vi "Compose TOML String.vi"(8 "error in (no error)":errorcluster, 11 "Value":T1) -> (0 "error out":errorcluster, 3 "String":string)   [LabVIEW 2019, in "BlueTOMLSerializer.lvlib"]
uses:
  BlueTOMLSerializer.lvlib
  TOML Value.ctl
  Compose Data.ctl
  Value.ctl
  Value Type.ctl
  Key-Value Pair.ctl
  <vilib>/regexp/Match Regular Expression.xnode
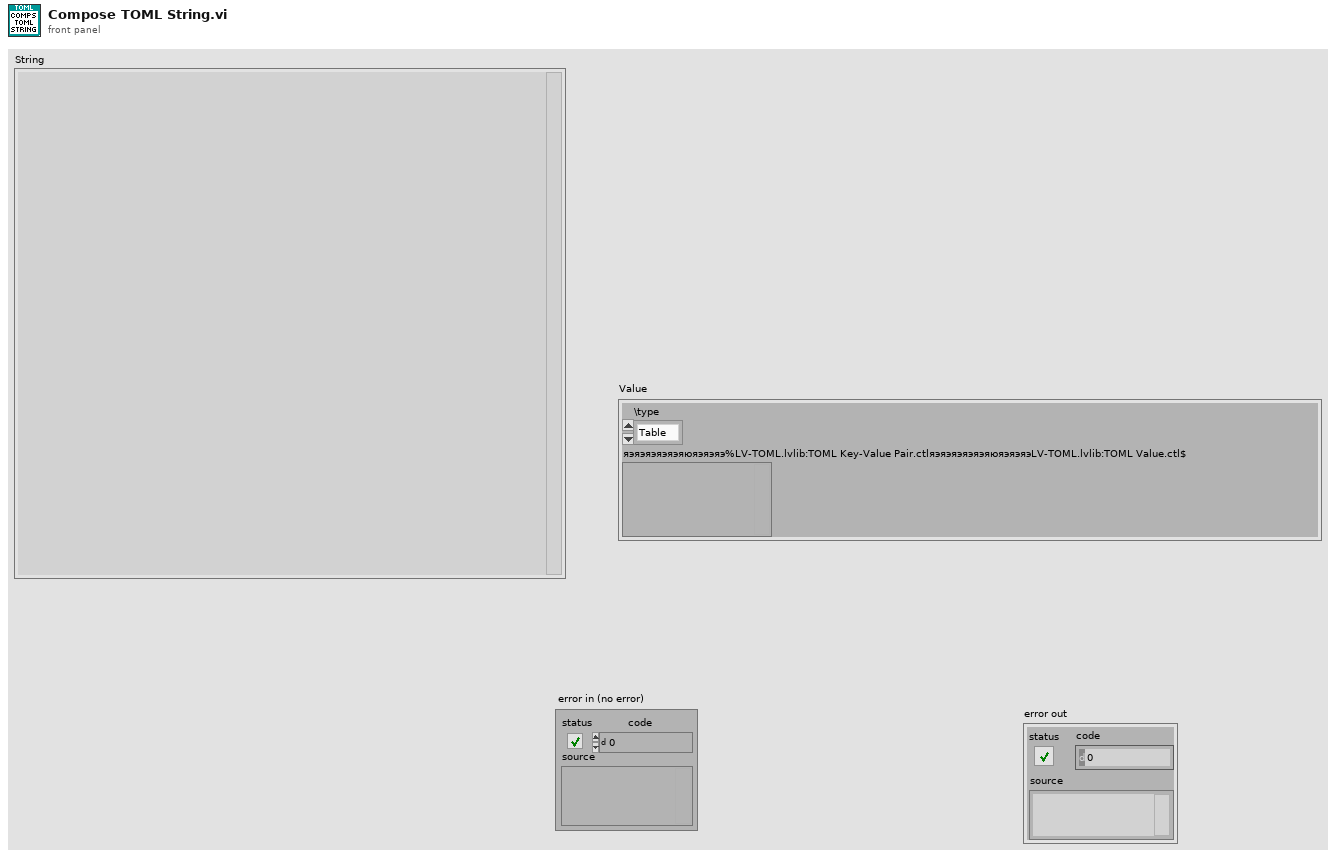
[diagram p1: front panel]
types:
  T1 = typedef "BlueTOMLSerializer.lvlib/TOML Value.ctl" = cluster{"\\type":enum16{"Table", "Array", "String", "Integer", "Float", "Boolean", "Offset Date-Time", "Local Date-Time", "Local Date", "Local Time"}, "яэяэяэяэяэяюяэяэяэ%LV-TOML.lvlib:TOML Key-Value Pair.ctlяэяэяэяэяэяюяэяэяэLV-TOML.lvlib:TOML Value.ctl$":variant}
  T2 = typedef "BlueTOMLSerializer.lvlib/Compose Data.ctl" = cluster{"Value":T3, "Prepend":string, "Append":string, "Inline":bool, "Name":string}
  T3 = typedef "BlueTOMLSerializer.lvlib/Value.ctl" = cluster{"Type":T4, "Value":variant}
  T4 = typedef "BlueTOMLSerializer.lvlib/Value Type.ctl" = enum16{"Table", "Array", "String", "Integer", "Float", "Boolean", "Offset Date-Time", "Local Date-Time", "Local Date", "Local Time"}
  T5 = typedef "BlueTOMLSerializer.lvlib/Key-Value Pair.ctl" = cluster{"Key":string, "Value":T3}
  T6 = enum16{"Table", "Array", "String", "Integer", "Float", "Boolean", "Offset Date-Time", "Local Date-Time", "Local Date", "Local Time"}
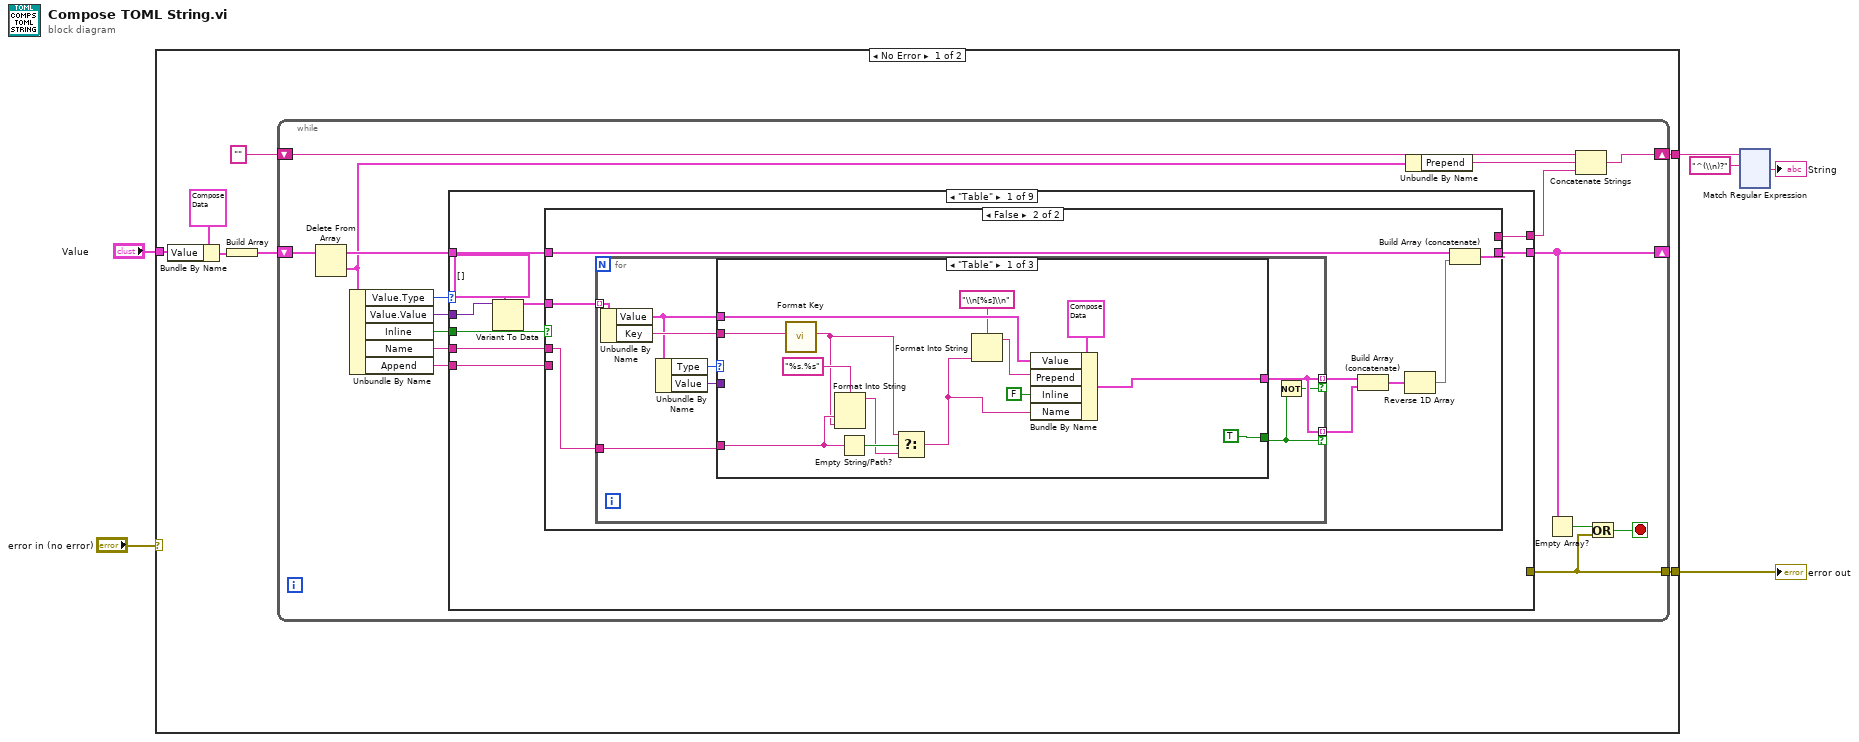
[diagram p0: block diagram]
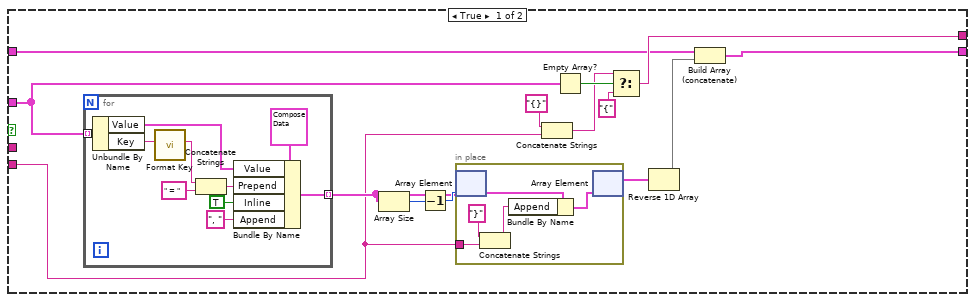
[diagram p2: hidden frame]
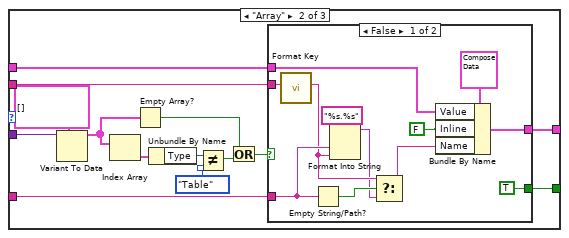
[diagram p3: hidden frame]
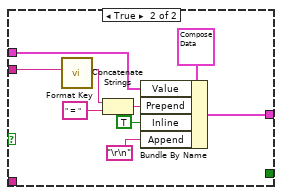
[diagram p4: hidden frame]
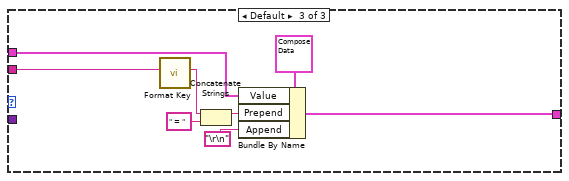
[diagram p5: hidden frame]
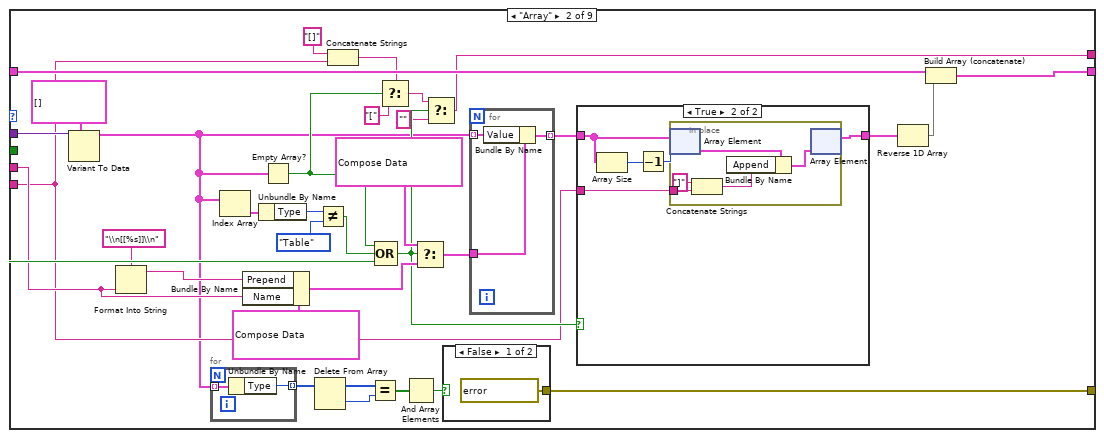
[diagram p6: hidden frame]
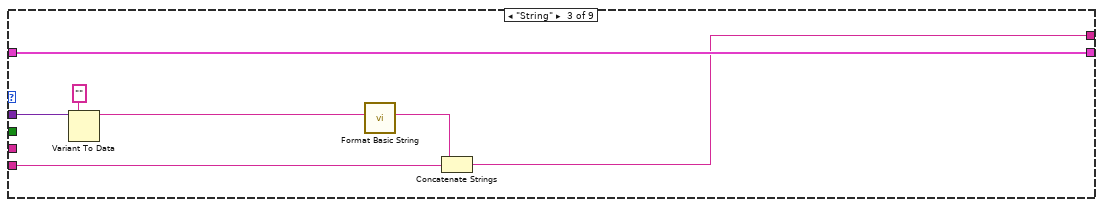
[diagram p9: hidden frame]
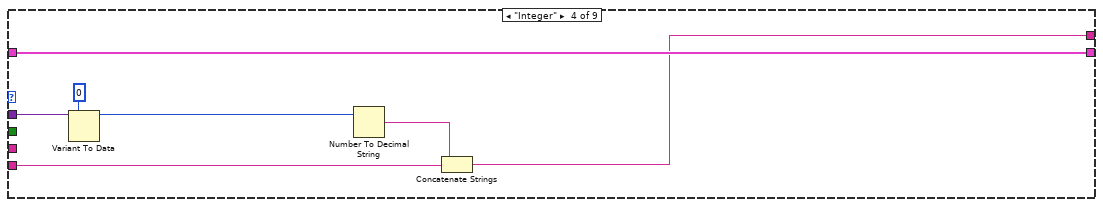
[diagram p10: hidden frame]
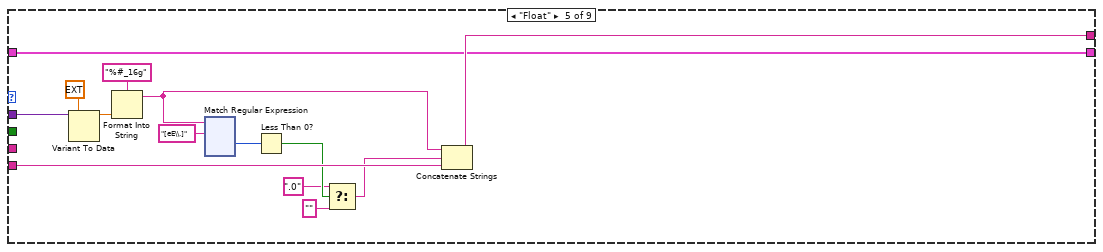
[diagram p11: hidden frame]
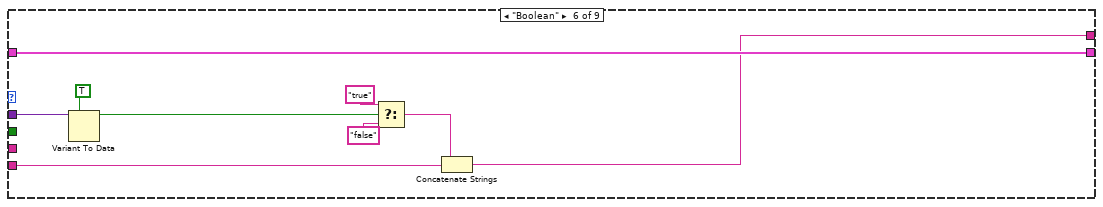
[diagram p12: hidden frame]
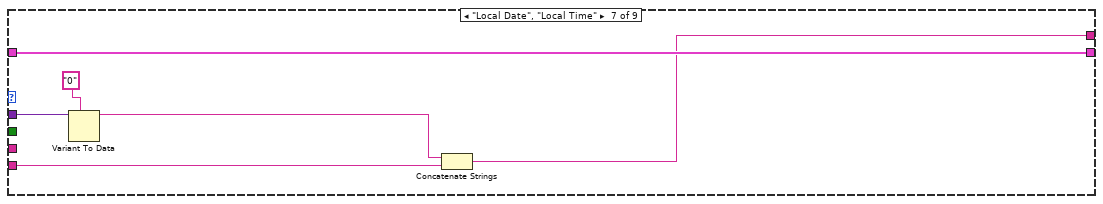
[diagram p13: hidden frame]
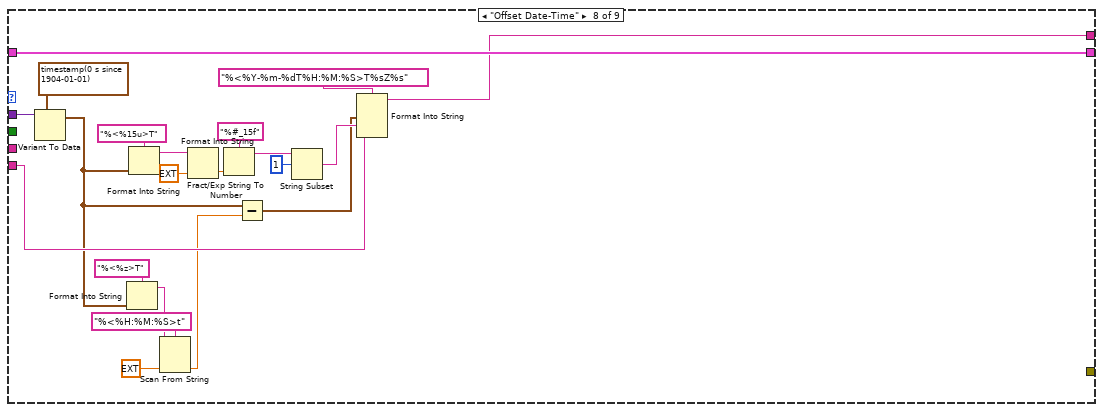
[diagram p14: hidden frame]
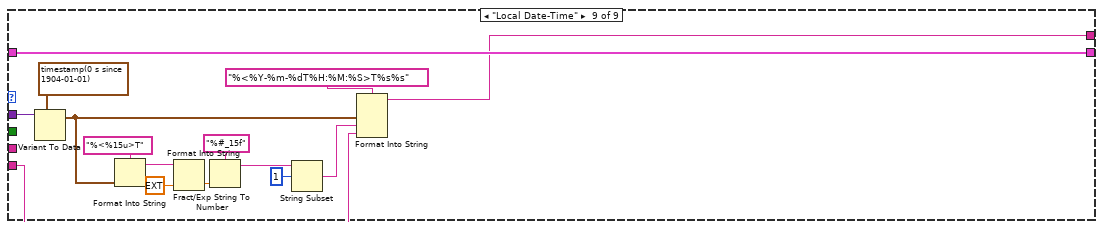
[diagram p15: hidden frame]
diagram:
  n1 = case shown="No Error" "error in (no error)" {
    selector: "error in (no error)" -> [_ w387]
    tunnel: "Value" -> [w10 _]
    tunnel: [w8 _] -> w1
    tunnel: [w7 w387] -> w4
    frame No Error {
      n2 = Bundle By Name(cluster=T2 {"Value"={"Type"=enum."Table", "Value"=variant}, "Prepend"="", "Append"="", "Inline"=FALSE, "Name"=""}, "Value"=w10) -> (w9:T2)
      n3 = Build Array(w9) -> (w12:T2[])
      n4 = while {
        shift-right: [w20] -> w8
        shift-left: "" -> [w23]
        shift-right: [w21] -> _
        shift-left: w12 -> [w29]
        tunnel: [w14] -> w7
        stop <- w15 stop-if-true
        n5 = Delete From Array(array=w29) -> (deleted portion=w18:T2, array with subset deleted=w26:T2[])  [unwired: 2 in]
        n6 = Unbundle By Name(w18) -> ("Value.Type"=w28:T4, "Value.Value"=w27:variant, "Inline"=w25:bool, "Name"=w24:string, "Append"=w16:string)
        n7 = case shown="\"Table\"" w28 {
          tunnel: w27 -> [w35 w176 w199 w206 w221 w344 w350 w370 w385]
          tunnel: w26 -> [w38 w163 w200 w207 w216 w342 w348 w371 w386]
          tunnel: [w37 w149 w200 w207 w216 w342 w348 w371 w386] -> w21
          tunnel: w25 -> [w36 w170 _ _ _ _ _ _ _]
          tunnel: w24 -> [w32 w152 _ _ _ _ _ _ _]
          tunnel: [w30 w156 w194 w201 w218 w336 w345 w362 w379] -> w19
          tunnel: w16 -> [w31 w150 w195 w204 w219 w343 w349 w363 w380]
          tunnel: [_ w142 _ _ _ _ _ _ _] -> w14
          frame "Table" {
            n8 = Variant To Data(type=T5[] [], Variant=w35) -> (data=w33:T5[])  [unwired: 1 in, 1 out]
            n9 = case shown="False" w36 {
              tunnel: w38 -> [w42 w75]
              tunnel: [w41 w74] -> w37
              tunnel: w33 -> [w49 w71]
              tunnel: w32 -> [_ w73]
              tunnel: w31 -> [w46 _]
              tunnel: [w45 _] -> w30
              frame True {
                n10 = for {
                  tunnel: w49 -> [w67] mode=indexing
                  tunnel: [w59] -> w50 mode=indexing
                  n11 = Unbundle By Name(w67) -> ("Value"=w64:T3, "Key"=w66:string)
                  n12 = call "Format Key.vi"("Key String"=w66) -> ("Formatted Key"=w62:string)  [unwired: 10 in]
                  n13 = Concatenate Strings(w62, " = " ("string")) -> (w63:string)
                  n14 = Bundle By Name(cluster=T2 {"Value"={"Type"=enum."Table", "Value"=variant}, "Prepend"="", "Append"="", "Inline"=FALSE, "Name"=""}, "Value"=w64, "Prepend"=w63, "Inline"=TRUE, "Append"=", ") -> (w59:T2)
                }
                n15 = Array Size(array=w50) -> (size(s)=w52:i32)
                n16 = Decrement(x=w52) -> (x-1=w51:i32)
                n17 = in-place {
                  in-place-border: w46 -> [w53]
                  n18 = in-place-array #1(w50, w51) -> (w57:T2)
                  n19 = Concatenate Strings("}" ("Prepend"), w53) -> (w54:string)
                  n20 = Bundle By Name(cluster=w57, "Append"=w54) -> (w56:T2)
                  n21 = in-place-array #1(w56) -> (w44:T2[])  [unwired: 1 out]
                }
                n22 = Concatenate Strings("{}" ("Prepend"), w46) -> (w39:string)
                n23 = Empty Array?(array=w49) -> (empty?=w48:bool)
                n24 = Select(t=w39, s=w48, f="{" ("t")) -> (s? t:f=w45:string)
                n25 = Reverse 1D Array(array=w44) -> (reversed array=w43:T2[])
                n26 = Build Array (concatenate)(w42, w43) -> (w41:T2[])
              }
              frame False {
                n27 = for {
                  tunnel: w71 -> [w84] mode=indexing
                  tunnel: [w78] -> w69 mode=indexing if=w77
                  tunnel: w73 -> [w80]
                  tunnel: [w78] -> w68 mode=indexing if=w76
                  n28 = Unbundle By Name(w84) -> ("Value"=w82:T3, "Key"=w83:string)
                  n29 = Unbundle By Name(w82) -> ("Type"=w81:T4, "Value"=w79:variant)
                  n30 = case shown="\"Table\"" w81 {
                    tunnel: w83 -> [w98 w112 w137]
                    tunnel: [w95 w111 w134] -> w78
                    tunnel: w82 -> [w94 w110 w136]
                    tunnel: w80 -> [w90 w109 _]
                    tunnel: w79 -> [_ w101 _]
                    tunnel: [TRUE w99 _] -> w76
                    frame "Table" {
                      n31 = call "Format Key.vi"("Key String"=w98) -> ("Formatted Key"=w88:string)  [unwired: 10 in]
                      n32 = Format Into String(format string="%s.%s", w90, w88) -> (resulting string=w87:string)  [unwired: 2 in, 1 out]
                      n33 = Empty String/Path?(string/path=w90) -> (empty?=w89:bool)
                      n34 = Select(t=w88, s=w89, f=w87) -> (s? t:f=w86:string)
                      n35 = Format Into String(format string="\\n[%s]\\n", w86) -> (resulting string=w91:string)  [unwired: 2 in, 1 out]
                      n36 = Bundle By Name(cluster=T2 {"Value"={"Type"=enum."Table", "Value"=variant}, "Prepend"="", "Append"="", "Inline"=FALSE, "Name"=""}, "Value"=w94, "Prepend"=w91, "Inline"=FALSE, "Name"=w86) -> (w95:T2)
                    }
                    frame "Array" {
                      n37 = Variant To Data(type=T3[] [], Variant=w101) -> (data=w104:T3[])  [unwired: 1 in, 1 out]
                      n38 = Index Array(array=w104) -> (element=w106:T3)  [unwired: 1 in]
                      n39 = Empty Array?(array=w104) -> (empty?=w108:bool)
                      n40 = Unbundle By Name(w106) -> ("Type"=w105:T4)
                      n41 = Not Equal?(x=w105, y=T6."Table") -> (x != y?=w107:bool)
                      n42 = Or(x=w108, y=w107) -> (x .or. y?=w100:bool)
                      n43 = case shown="False" w100 {
                        tunnel: w112 -> [w119 w127]
                        tunnel: [w122 w125] -> w111
                        tunnel: w110 -> [w121 w128]
                        tunnel: w109 -> [w118 _]
                        tunnel: [TRUE _] -> w99
                        frame False {
                          n44 = call "Format Key.vi"("Key String"=w119) -> ("Formatted Key"=w116:string)  [unwired: 10 in]
                          n45 = Empty String/Path?(string/path=w118) -> (empty?=w117:bool)
                          n46 = Format Into String(format string="%s.%s", w118, w116) -> (resulting string=w115:string)  [unwired: 2 in, 1 out]
                          n47 = Select(t=w116, s=w117, f=w115) -> (s? t:f=w114:string)
                          n48 = Bundle By Name(cluster=T2 {"Value"={"Type"=enum."Table", "Value"=variant}, "Prepend"="", "Append"="", "Inline"=FALSE, "Name"=""}, "Value"=w121, "Inline"=FALSE, "Name"=w114) -> (w122:T2)
                        }
                        frame True {
                          n49 = call "Format Key.vi"("Key String"=w127) -> ("Formatted Key"=w131:string)  [unwired: 10 in]
                          n50 = Concatenate Strings(w131, " = " ("string")) -> (w132:string)
                          n51 = Bundle By Name(cluster=T2 {"Value"={"Type"=enum."Table", "Value"=variant}, "Prepend"="", "Append"="", "Inline"=FALSE, "Name"=""}, "Value"=w128, "Prepend"=w132, "Inline"=TRUE, "Append"="\r\n") -> (w125:T2)
                        }
                      }
                    }
                    frame Default {
                      n52 = call "Format Key.vi"("Key String"=w137) -> ("Formatted Key"=w139:string)  [unwired: 10 in]
                      n53 = Concatenate Strings(w139, " = " ("string")) -> (w140:string)
                      n54 = Bundle By Name(cluster=T2 {"Value"={"Type"=enum."Table", "Value"=variant}, "Prepend"="", "Append"="", "Inline"=FALSE, "Name"=""}, "Value"=w136, "Prepend"=w140, "Append"="\r\n") -> (w134:T2)
                    }
                  }
                  n55 = Not(x=w76) -> (.not. x?=w77:bool)
                }
                n56 = Build Array (concatenate)(w69, w68) -> (w70:T2[])
                n57 = Reverse 1D Array(array=w70) -> (reversed array=w72:T2[])
                n58 = Build Array (concatenate)(w75, w72) -> (w74:T2[])
              }
            }
          }
          frame "Array" {
            n59 = Variant To Data(type=T3[] [], Variant=w176) -> (data=w148:T3[])  [unwired: 1 in, 1 out]
            n60 = Format Into String(format string="\\n[[%s]]\\n", w152) -> (resulting string=w153:string)  [unwired: 2 in, 1 out]
            n61 = for {
              tunnel: w148 -> [w179] mode=indexing
              tunnel: [w178] -> w147 mode=indexing
              n62 = Unbundle By Name(w179) -> ("Type"=w178:T4)
            }
            n63 = Index Array(array=w148) -> (element=w174:T3)  [unwired: 1 in]
            n64 = Bundle By Name(cluster=T2 {"Value"={"Type"=enum."Table", "Value"=variant}, "Prepend"="", "Append"="", "Inline"=FALSE, "Name"=""}, "Prepend"=w153, "Name"=w152) -> (w167:T2)
            n65 = Unbundle By Name(w174) -> ("Type"=w173:T4)
            n66 = Empty Array?(array=w148) -> (empty?=w160:bool)
            n67 = Delete From Array(array=w147) -> (deleted portion=w145:T4, array with subset deleted=w146:T4[])  [unwired: 2 in]
            n68 = Not Equal?(x=w173, y=T6."Table") -> (x != y?=w171:bool)
            n69 = Concatenate Strings("[]", w150) -> (w158:string)
            n70 = Equal?(x=w146, y=w145) -> (x = y?=w144:bool[])
            n71 = Compound Arithmetic op=OR(w160, w171, w170) -> (w157:bool)
            n72 = Select(t=w158, s=w160, f="[") -> (s? t:f=w155:string)
            n73 = And Array Elements(Boolean array=w144) -> (logical AND=w143:bool)
            n74 = Select(t=T2 {"Value"={"Type"=enum."Table", "Value"=variant}, "Prepend"="", "Append"=", ", "Inline"=TRUE, "Name"=""} ("cluster"), s=w157, f=w167) -> (s? t:f=w166:T2)
            n75 = Select(t=w155, s=w157, f="") -> (s? t:f=w156:string)
            n76 = case shown="False" w143 {
              tunnel: [errorcluster {"status"=TRUE, "code"=5001, "source"="Array elements must all have same type"} ("error constant") _] -> w142
              frame False {
              }
              frame True {
              }
            }
            n77 = for {
              tunnel: w148 -> [w193] mode=indexing
              tunnel: w166 -> [w192]
              tunnel: [w191] -> w165 mode=indexing
              n78 = Bundle By Name(cluster=w192, "Value"=w193) -> (w191:T2)
            }
            n79 = case shown="True" w157 {
              tunnel: w165 -> [w180 w182]
              tunnel: [w180 w183] -> w164
              tunnel: w150 -> [_ w181]
              frame False {
              }
              frame True {
                n80 = Array Size(array=w182) -> (size(s)=w185:i32)
                n81 = Decrement(x=w185) -> (x-1=w184:i32)
                n82 = in-place {
                  in-place-border: w181 -> [w186]
                  n83 = in-place-array #2(w182, w184) -> (w190:T2)
                  n84 = Concatenate Strings("]" ("string"), w186) -> (w188:string)
                  n85 = Bundle By Name(cluster=w190, "Append"=w188) -> (w189:T2)
                  n86 = in-place-array #2(w189) -> (w183:T2[])  [unwired: 1 out]
                }
              }
            }
            n87 = Reverse 1D Array(array=w164) -> (reversed array=w162:T2[])
            n88 = Build Array (concatenate)(w163, w162) -> (w149:T2[])
          }
          frame "String" {
            n89 = Variant To Data(type="", Variant=w199) -> (data=w197:string)  [unwired: 1 in, 1 out]
            n90 = call "Format Basic String.vi"("String"=w197) -> ("Formatted Basic String"=w196:string)  [unwired: 10 in]
            n91 = Concatenate Strings(w196, w195) -> (w194:string)
          }
          frame "Integer" {
            n92 = Variant To Data(type=i64 0, Variant=w206) -> (data=w203:i64)  [unwired: 1 in, 1 out]
            n93 = Number To Decimal String(number=w203) -> (decimal integer string=w202:string)  [unwired: 1 in]
            n94 = Concatenate Strings(w202, w204) -> (w201:string)
          }
          frame "Float" {
            n95 = Variant To Data(type=ext 0.0, Variant=w221) -> (data=w217:ext)  [unwired: 1 in, 1 out]
            n96 = Format Into String(format string="%#_16g", w217) -> (resulting string=w211:string)  [unwired: 2 in, 1 out]
            n97 = xnode "Match Regular Expression"("input string"=w211, "regular expression"="[eE\\.]") -> ("offset past match"=w213:i32)  [unwired: 4 in, 4 out]
            n98 = Less Than 0?(x=w213) -> (x < 0?=w212:bool)
            n99 = Select(t=".0", s=w212, f="") -> (s? t:f=w208:string)
            n100 = Concatenate Strings(w211, w208, w219) -> (w218:string)
          }
          frame "Boolean" {
            n101 = Variant To Data(type=TRUE, Variant=w344) -> (data=w340:bool)  [unwired: 1 in, 1 out]
            n102 = Select(t="true", s=w340, f="false") -> (s? t:f=w337:string)
            n103 = Concatenate Strings(w337, w343) -> (w336:string)
          }
          frame "Local Date", "Local Time" {
            n104 = Variant To Data(type="0", Variant=w350) -> (data=w346:string)  [unwired: 1 in, 1 out]
            n105 = Concatenate Strings(w346, w349) -> (w345:string)
          }
          frame "Offset Date-Time" {
            n106 = Variant To Data(type=timestamp(0 s since 1904-01-01), Variant=w370) -> (data=w352:timestamp)  [unwired: 1 in, 1 out]
            n107 = Format Into String(format string="%<%z>T", w352) -> (resulting string=w355:string)  [unwired: 2 in, 1 out]
            n108 = Format Into String(format string="%<%15u>T", w352) -> (resulting string=w360:string)  [unwired: 2 in, 1 out]
            n109 = Scan From String(format string="%<%H:%M:%S>t", input string=w355, default 1=ext 0.0 ("default value 1")) -> (output 1=w353:ext)  [unwired: 2 in, 3 out]
            n110 = Fract/Exp String To Number(string=w360, default (0 dbl)=ext 0.0 ("default (0 DBL)")) -> (number=w358:ext)  [unwired: 2 in, 1 out]
            n111 = Format Into String(format string="%#_15f", w358) -> (resulting string=w367:string)  [unwired: 2 in, 1 out]
            n112 = Subtract(x=w352, y=w353) -> (x-y=w351:timestamp)
            n113 = String Subset(string=w367, offset (0)=1) -> (substring=w364:string)  [unwired: 1 in]
            n114 = Format Into String(format string="%<%Y-%m-%dT%H:%M:%S>T%sZ%s", w351, w364, w363) -> (resulting string=w362:string)  [unwired: 2 in, 1 out]
          }
          frame "Local Date-Time" {
            n115 = Variant To Data(type=timestamp(0 s since 1904-01-01), Variant=w385) -> (data=w372:timestamp)  [unwired: 1 in, 1 out]
            n116 = Format Into String(format string="%<%15u>T", w372) -> (resulting string=w376:string)  [unwired: 2 in, 1 out]
            n117 = Fract/Exp String To Number(string=w376, default (0 dbl)=ext 0.0 ("default (0 DBL)")) -> (number=w374:ext)  [unwired: 2 in, 1 out]
            n118 = Format Into String(format string="%#_15f", w374) -> (resulting string=w373:string)  [unwired: 2 in, 1 out]
            n119 = String Subset(string=w373, offset (0)=1) -> (substring=w381:string)  [unwired: 1 in]
            n120 = Format Into String(format string="%<%Y-%m-%dT%H:%M:%S>T%s%s", w372, w381, w380) -> (resulting string=w379:string)  [unwired: 2 in, 1 out]
          }
        }
        n121 = Unbundle By Name(w18) -> ("Prepend"=w17:string)
        n122 = Empty Array?(array=w21) -> (empty?=w22:bool)
        n123 = Concatenate Strings(w23, w17, w19) -> (w20:string)
        n124 = Or(x=w22, y=w14) -> (x .or. y?=w15:bool)
      }
    }
    frame Error {
    }
  }
  "error out" <- w4
  n125 = xnode "Match Regular Expression"("input string"=w1, "regular expression"="^(\\n)?") -> ("after match"=→"String":string)  [unwired: 4 in, 4 out]
